vi "Stop Core.vi"(10 "final error code":i32, 11 "Mediator In":refnum<class "IMediator.lvclass">) -> (3 "Mediator Out":refnum<class "IMediator.lvclass">)   [LabVIEW 2018, in "MVA Framework.lvlib" / "IMediator.lvlib" / "IMediator.lvclass"]
doc: "(<B>Filename</B>: Actor Framework.lvlib:Actor.lvclass:Stop Core.vi)\n\nDefines what the actor does before it stops. Use the <B>final error code</B> input to determine whether the actor shut down in response to an error.\n\nBy default, this method does nothing. A descendant class may override it to define behavior, such as shutting down any processes the actor initiated in its override of the Actor Core method."
uses:
  IMediator.lvclass
  <vilib>/ActorFramework/Actor/Actor.lvclass
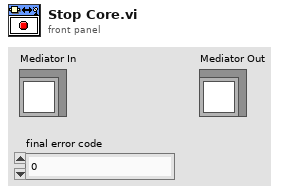
[diagram p1: front panel]
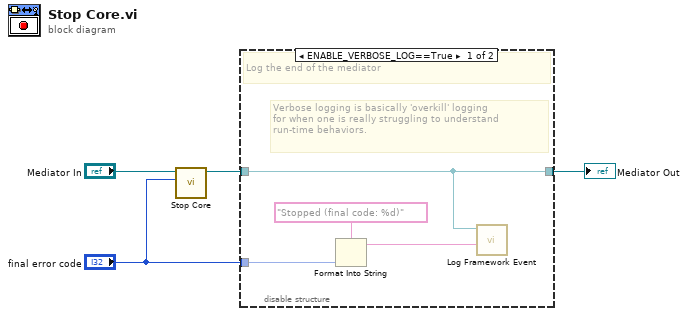
[diagram p0: block diagram]
diagram:
  n1 = call-parent "Stop Core.vi"("final error code"="final error code", "Actor in"="Mediator In") -> ("Actor out"=w3:refnum<class "IMediator.lvclass">)  [unwired: 9 in]
  n2 = disable-structure shown="ENABLE_VERBOSE_LOG==True" {
    disable-tunnel: w3 -> [w5 w9]
    disable-tunnel: [w5 w9] -> w2
    disable-tunnel: "final error code" -> [w8 _]
    frame condition #0 {
      # "Verbose logging is basically 'overkill' logging\nfor when one is really struggling to understand\nrun-time behaviors."
      # "Log the end of the mediator"
      n3 = Format Into String(format string="Stopped (final code: %d)", w8) -> (resulting string=w6:string)  [unwired: 2 in, 1 out]
      n4 = call "Log Framework Event.vi"("Data To Log"=w6, "IMediator In"=w5) -> ()  [unwired: 9 in, 1 out]
    }
    frame condition #1 (active) {
      # "Remove all logging from this method at compile time"
    }
  }
  "Mediator Out" <- w2
